vi "MC4_Sensor View Window.vi"(10 "SRV In":refnum<k5>, 11 "Sensors Config File Path":path) -> (0 "error out":errorcluster)   [LabVIEW 2009]
doc: "Save a renamed copy of this template to a location of your choice. Set \"Sensor Window Filepath\" in your System Config to point to your copy of the Sensor Window.\n\nSet \"Make All Visible\" (located just below the frame) to TRUE and run this VI directly from its own Run Arrow one time in order to make all the controls visible so that you can move controls around on the front panel. If there are sensors you will not be using, move them out of the frame off to the right.\n\nFrame should be 746x706. Check this by clicking arrow mouse over bottom right corner of frame. The window will resize to the frame at runtime.\n\nTo place IMAGE ON THE FRONT PANEL, go to Edit >> Import Picture to Clipboard (this works better in LabVIEW rather than copying to clipboard from another application). Then you can paste (Ctrl+V) the image on the front panel. It is recommended to then select your image and select Move To Back (Ctrl+Shift+J) so that sensors are on top if there is any overlap between sensors and your image.\n\n\nAuthor: Mike Schultz\n\nLogicPD, Inc\nwww.logicpd.com"
uses:
  SRV VIs/Sensors/SRV_Sensor View refs.ctl
  SRV VIs/Sensors/SRV_Sensor Config Cluster.ctl
  SRV VIs/Sensors/SRV_Sensor Analog-Digital.ctl
  SRV VIs/Sensors/SRV_Sensor Sampling Mode.ctl
  SRV VIs/Sensors/SRV_Sensor View Config Cluster.ctl
  SRV VIs/Sensors/SRV_Sensors Names.ctl
  SRV VIs/Sensors/SRV_Sensor PicoC Shared Var Type.ctl
  SRV VIs/Sensors/SRV_Sensor Config-Command Cluster.ctl
  SRV VIs/Support/SRV_Command-Data Queue Data Type.ctl
  SRV VIs/Sensors/SRV_Sensor-Value Cluster.ctl
  <vilib>/Utility/error.llb/DialogType.ctl
panel:
  in  "Make All Visible":bool
  out "Overflow Indicator":bool
  out "# elements in queue":i32
  out "Command":string
  in  "Poll":bool
  out "Boolean 32":bool
  out "Boolean 31":bool
  out "Boolean 30":bool
  out "Boolean 29":bool
  out "Boolean 28":bool
  out "Boolean 27":bool
  out "Boolean 26":bool
  out "Boolean 25":bool
  out "Boolean 24":bool
  out "Boolean 23":bool
  out "Boolean 22":bool
  out "Boolean 21":bool
  out "Boolean 20":bool
  out "Boolean 19":bool
  out "Boolean 18":bool
  out "Boolean 17":bool
  out "Boolean 16":bool
  out "Boolean 15":bool
  out "Boolean 14":bool
  out "Boolean 13":bool
  out "Boolean 12":bool
  out "Boolean 11":bool
  out "Boolean 10":bool
  out "Boolean 09":bool
  out "Boolean 08":bool
  out "Boolean 07":bool
  out "Boolean 06":bool
  out "Boolean 05":bool
  out "Boolean 04":bool
  out "Boolean 03":bool
  out "Boolean 02":bool
  out "Boolean 01":bool
  out "Numeric 08":dbl
  out "Numeric 07":dbl
  out "Numeric 06":dbl
  out "Numeric 05":dbl
  out "Numeric 04":dbl
  out "Numeric 03":dbl
  out "Numeric 02":dbl
  out "Numeric 01":dbl
  out "Meter 04":dbl(knob) scale=-1.0..0.0
  out "Meter 03":dbl(knob) scale=-1.0..0.0
  out "Meter 02":dbl(knob) scale=-1.0..0.0
  out "Meter 01":dbl(knob) scale=-1.0..0.0
  out "Gauge 04":dbl(knob) scale=-1.0..0.0
  out "Gauge 03":dbl(knob) scale=-1.0..0.0
  out "Gauge 02":dbl(knob) scale=-1.0..0.0
  out "Gauge 01":dbl(knob) scale=-1.0..0.0 scale format="%#.3g"
  # "SensorView Window"
  # "SensorPallet"
  # "SensorView Window Instructions\n\nUse the Arrow tool from the Tools Pallet to select, pull and place sensors into the SensorView Window. If you want to remove a sensor from the SensorView Window use the Arrow tool to select and pull the sensor back to the SensorPallet.\n\nTo open the Tools Pallet go to View/Tools Pallet in the standard tool bar. Be sure to close the Tools Pallet when you are finished creating your sensor dashboard.\n\n\n* BE SURE TO PLACE SENSORS BACK IN THEIR CORRECT LOCATION ON THE SENSORPALLET OR YOU WILL END UP WITH A MESS."
  # "Set to TRUE and run this VI directly from its own Run Arrow \none time in order to make all the controls visible so that \nyou can move controls around on the front panel.  If there \nare sensors you will not be using, move them out of the \nframe off to the right."
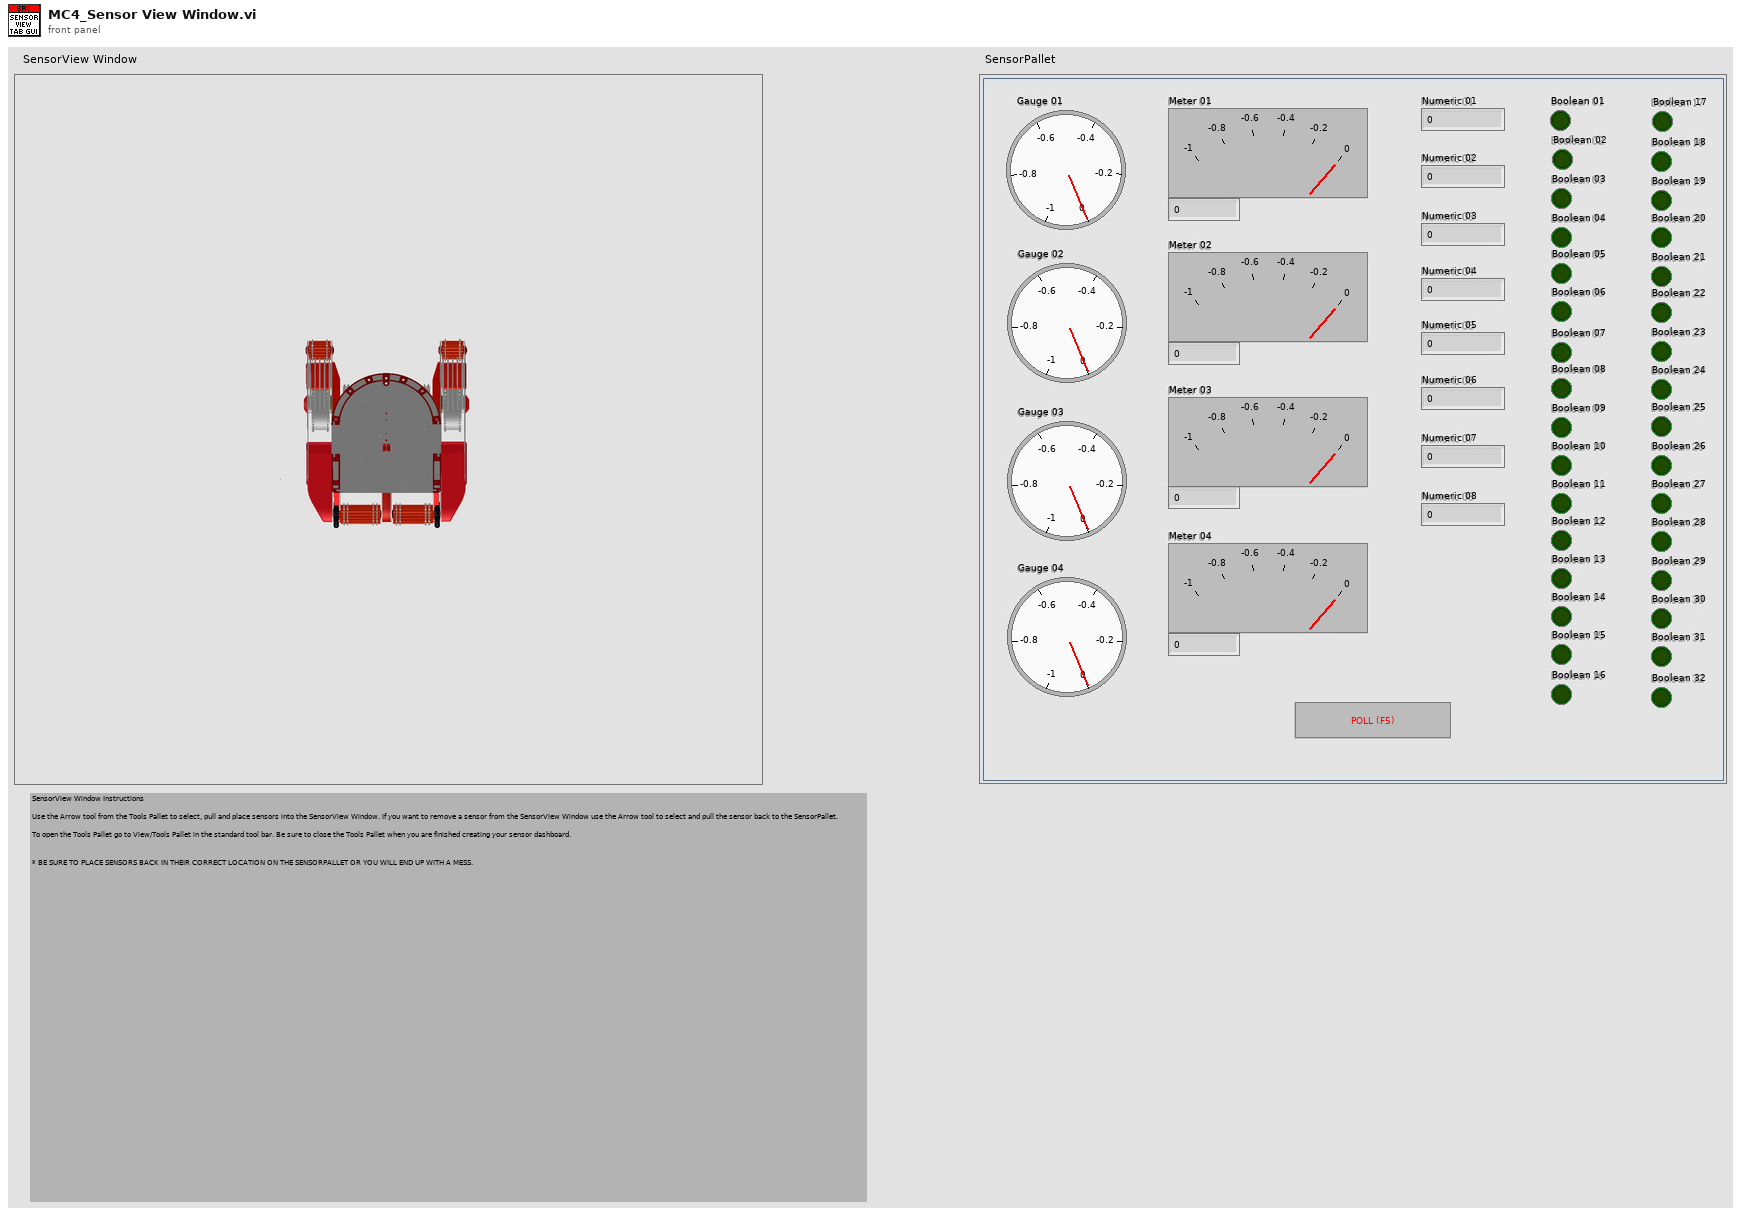
[diagram p1: front panel]
types:
  T1 = typedef "SRV_Command-Data Queue Data Type.ctl" = cluster{"Command":string, "Data":variant}
  T2 = typedef "SRV_Sensor View refs.ctl" = cluster{"Knob refs":refnum<vi>[], "Numeric refs":refnum<vi>[], "Boolean refs":refnum<vi>[]}
  T3 = typedef "SRV_Sensor Config Cluster.ctl" = cluster{"Name":string, "A/D":T4, "I2C Address":u8, "Register":u8, "Channel":u8, "Digital Mask":u8, "Units":string, "Sampling Mode":T5, "Sample Period (ms)":u32, "Formula":string, "Sensor View Config":T6, "Active":bool, "PicoC Shared Var Type":T8, "Index":u8, "Stream Multiple?":bool, "Index End":u8}
  T4 = typedef "SRV_Sensor Analog-Digital.ctl" = enum16{"Analog", "Digital", "RCMx1 Analog", "PicoC Shared"}
  T5 = typedef "SRV_Sensor Sampling Mode.ctl" = enum16{"Polled", "Streaming"}
  T6 = typedef "SRV_Sensor View Config Cluster.ctl" = cluster{"Sensor Name":T7, "Minimum":dbl, "Maximum":dbl}
  T7 = typedef "SRV_Sensors Names.ctl" = enum16{"Gauge 01", "Gauge 02", "Gauge 03", "Gauge 04", "Meter 01", "Meter 02", "Meter 03", "Meter 04", "Numeric 01", "Numeric 02", "Numeric 03", "Numeric 04", "Numeric 05", "Numeric 06", "Numeric 07", "Numeric 08", "Boolean 01", "Boolean 02", "Boolean 03", "Boolean 04", "Boolean 05", "Boolean 06", "Boolean 07", "Boolean 08", "Boolean 09", "Boolean 10", "Boolean 11", "Boolean 12", "Boolean 13", "Boolean 14", "Boolean 15", "Boolean 16", "Boolean 17", "Boolean 18", "Boolean 19", "Boolean 20", "Boolean 21", "Boolean 22", "Boolean 23", "Boolean 24", "Boolean 25", "Boolean 26", "Boolean 27", "Boolean 28", "Boolean 29", "Boolean 30", "Boolean 31", "Boolean 32"}
  T8 = typedef "SRV_Sensor PicoC Shared Var Type.ctl" = enum16{"String", "Integer", "Float"}
  T9 = typedef "SRV_Sensor Config-Command Cluster.ctl" = cluster{"Sensor Config":T3, "Command":string, "Constant Command":string}
  T10 = cluster{"user event":refnum<user-event>, "Version":string, "Sensor View refs":T2, "This VI ref":refnum<vi>, "Sensors Config File Path":path, "Sensors Config":T3[], "SRV ref":refnum<k5>, "Streaming Cfg-Cmds":T9[], "Polled Cfg-Cmds":T9[], "Off Cfg-Cmds":T9[], "Streaming Constant Commands":string[], "Polled Constant Commands":string[], "Make All Visible":bool}
  T11 = typedef "SRV_Sensor-Value Cluster.ctl" = cluster{"Sensor Name":T7, "Value":dbl}
  T12 = typedef "DialogType.ctl" = u16
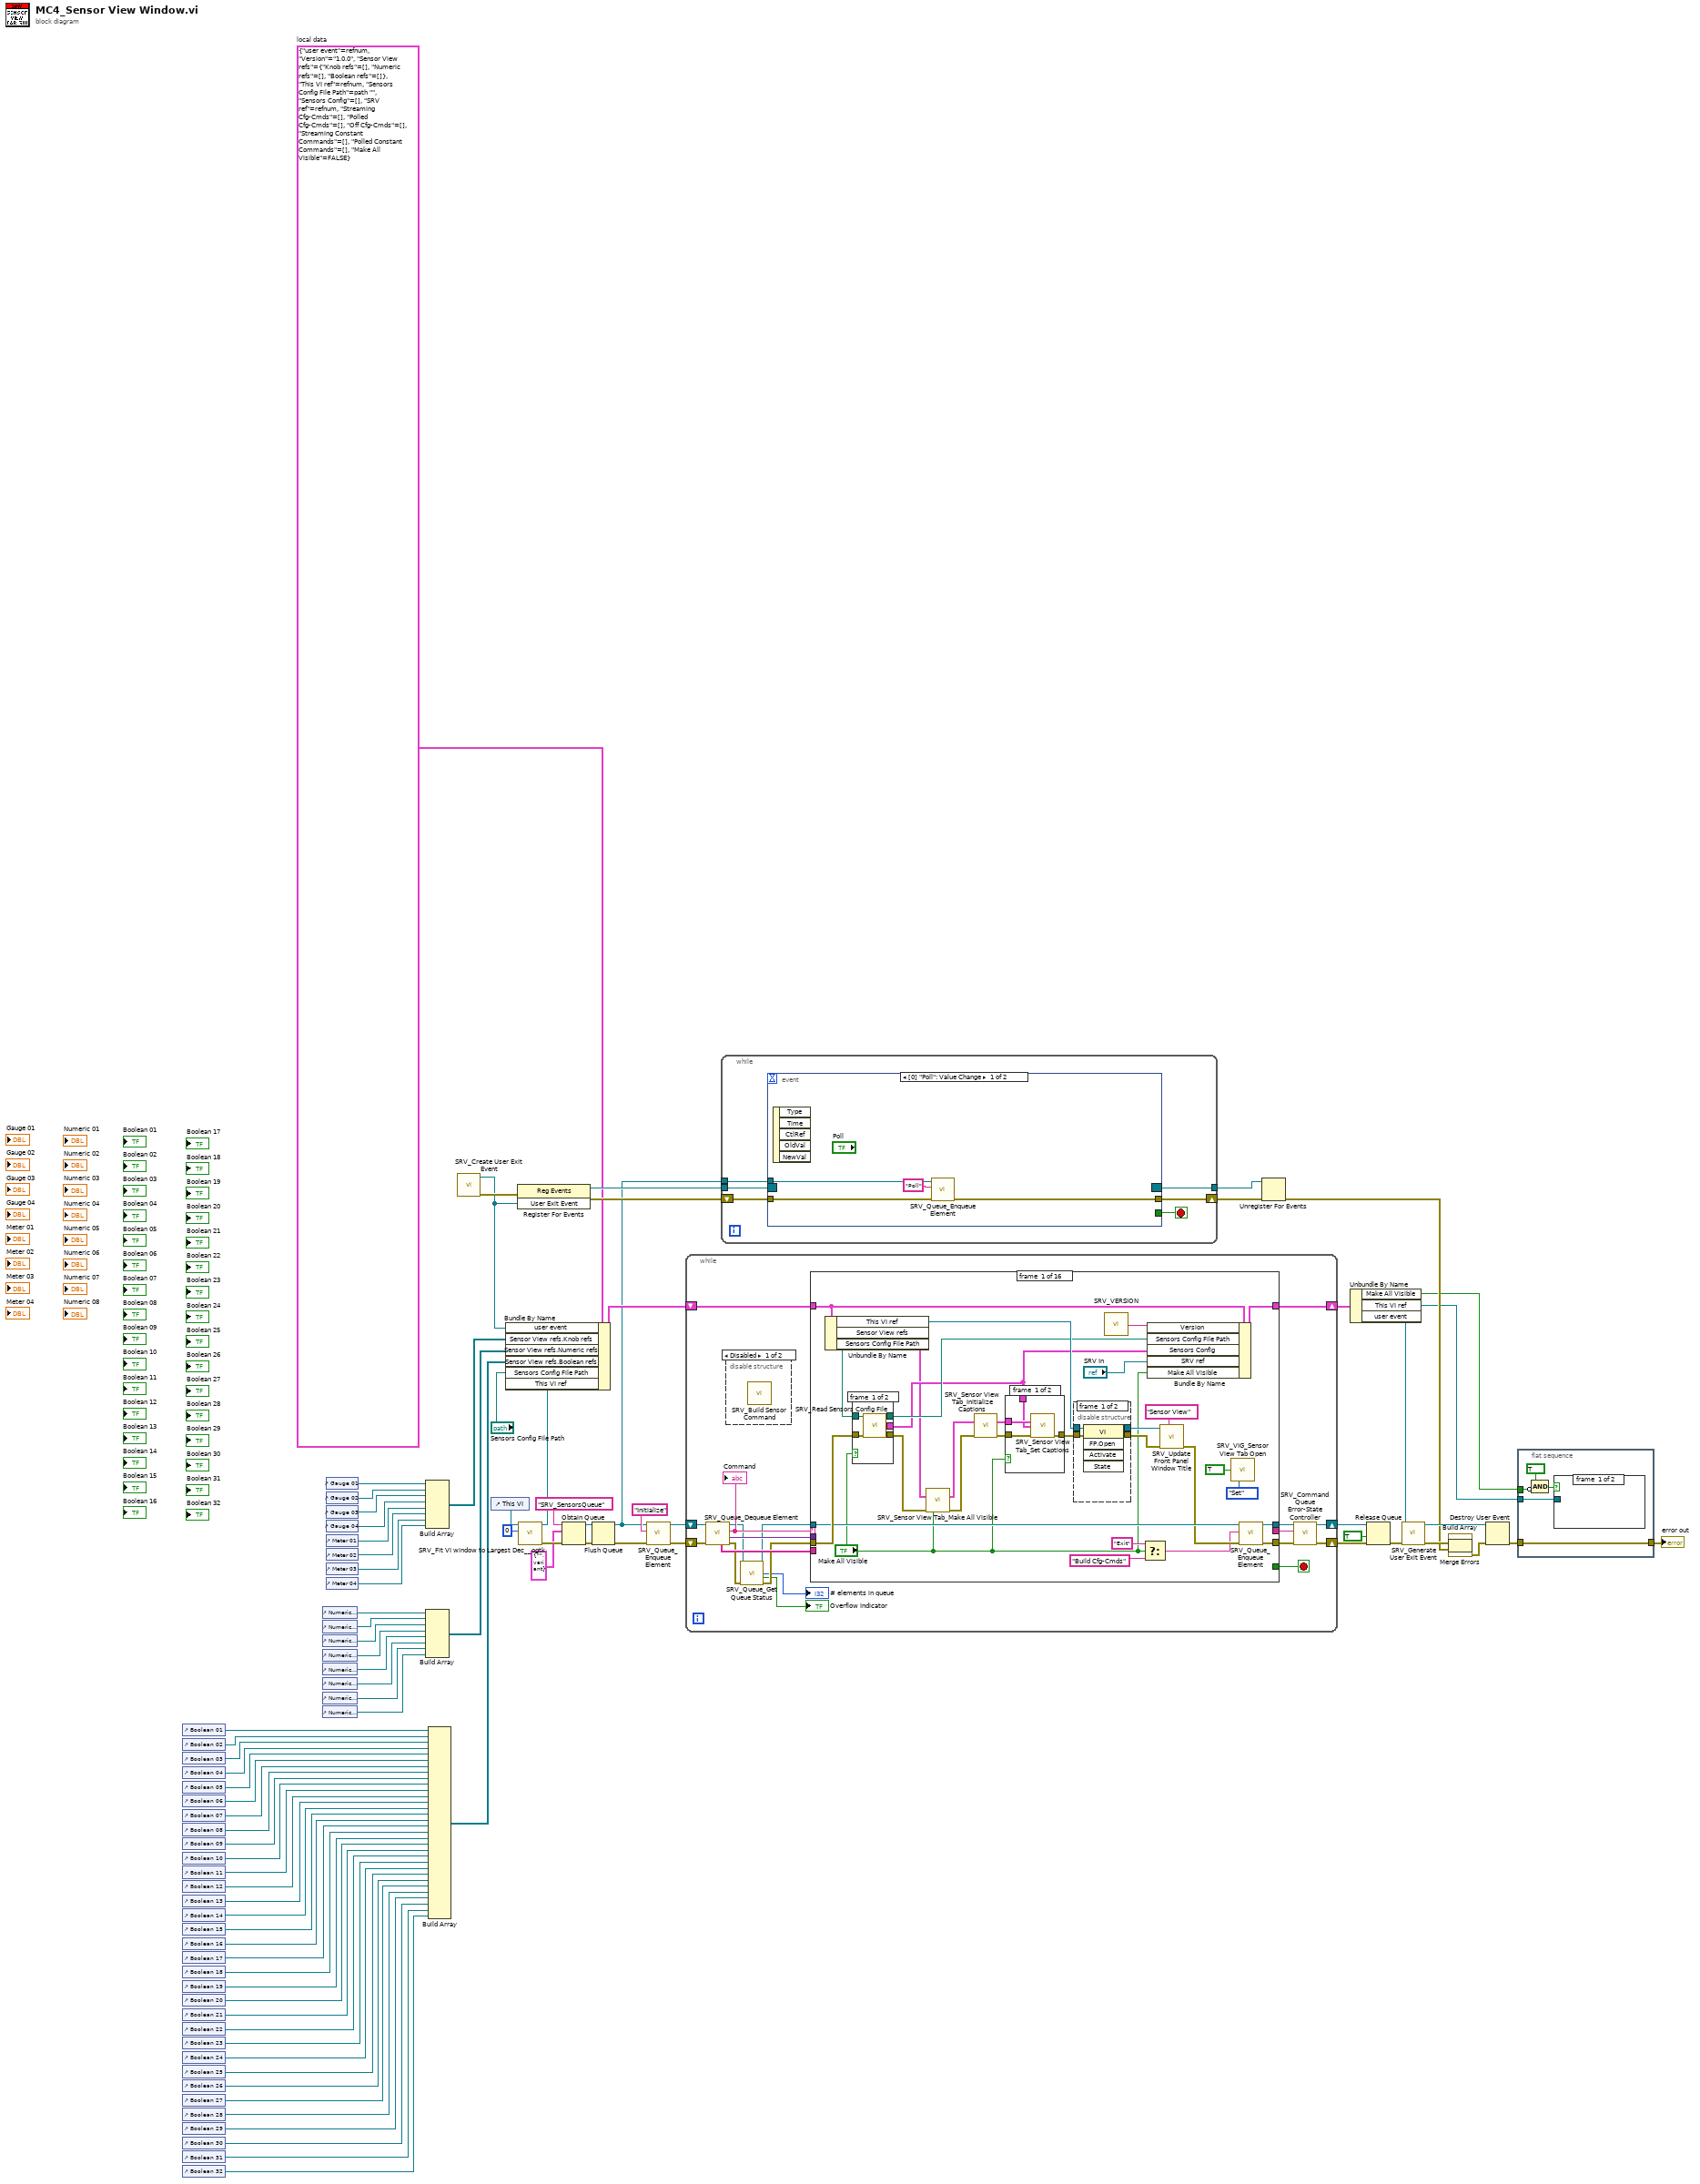
[diagram p0: block diagram]
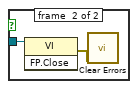
[diagram p2: hidden frame]
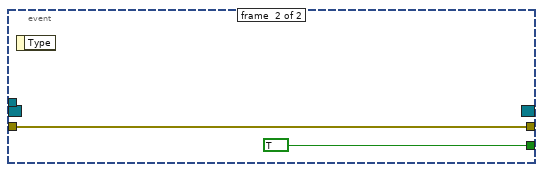
[diagram p3: hidden frame]
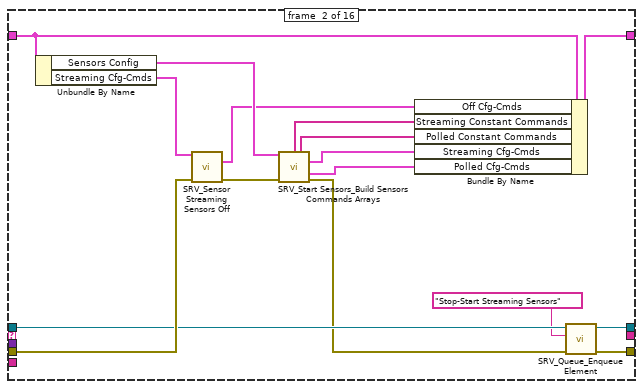
[diagram p8: hidden frame]
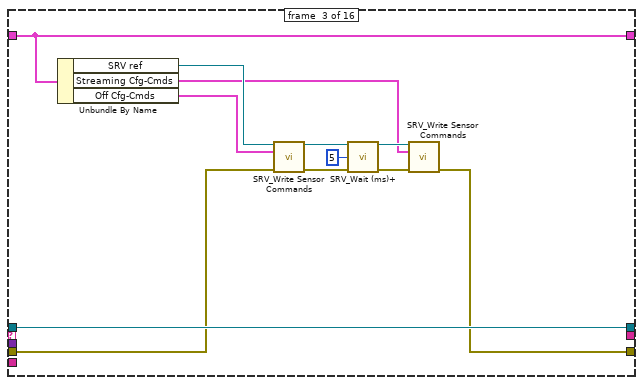
[diagram p9: hidden frame]
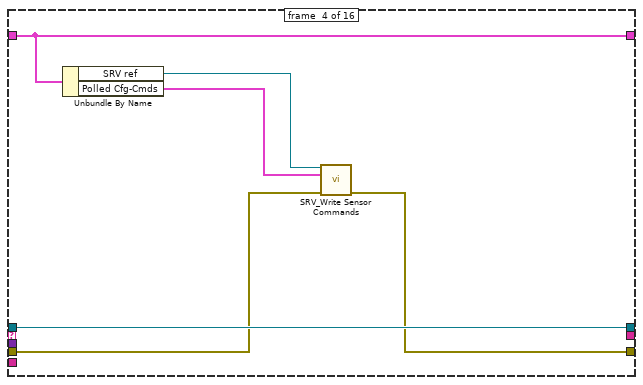
[diagram p10: hidden frame]
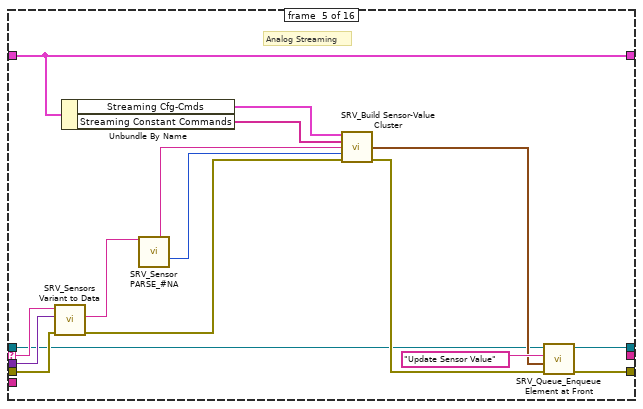
[diagram p11: hidden frame]
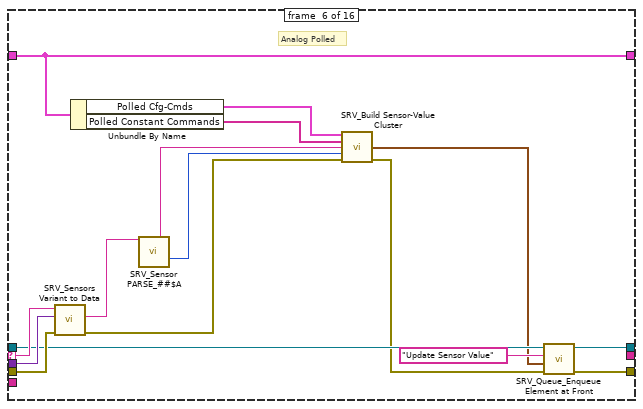
[diagram p12: hidden frame]
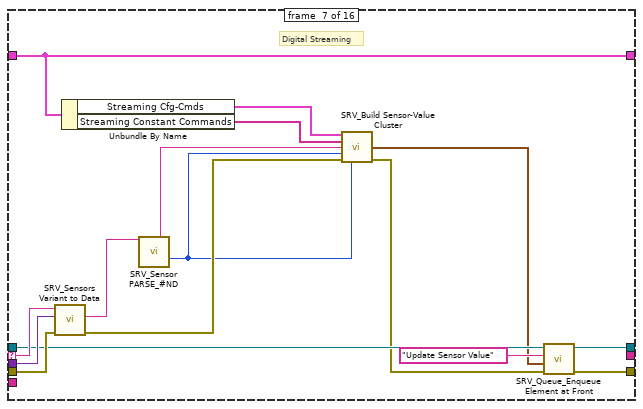
[diagram p13: hidden frame]
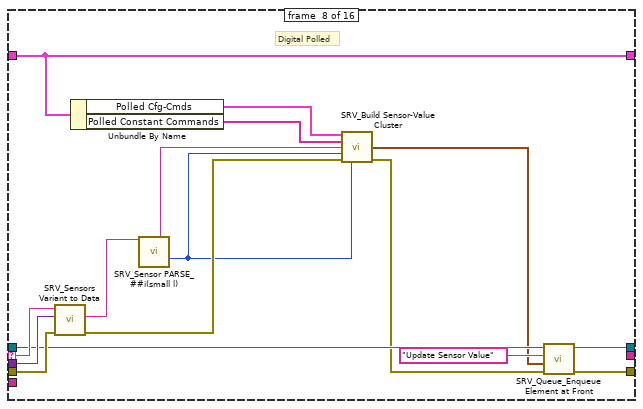
[diagram p14: hidden frame]
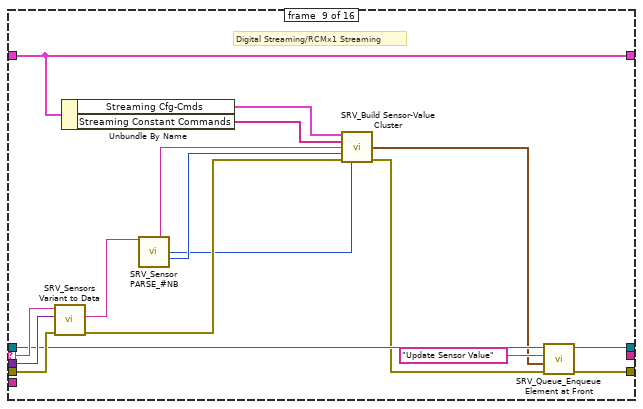
[diagram p15: hidden frame]
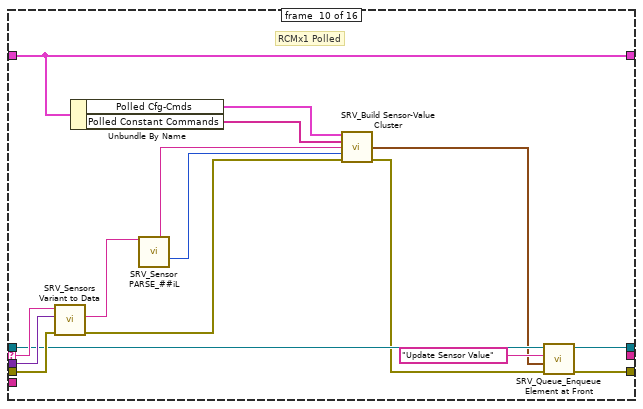
[diagram p16: hidden frame]
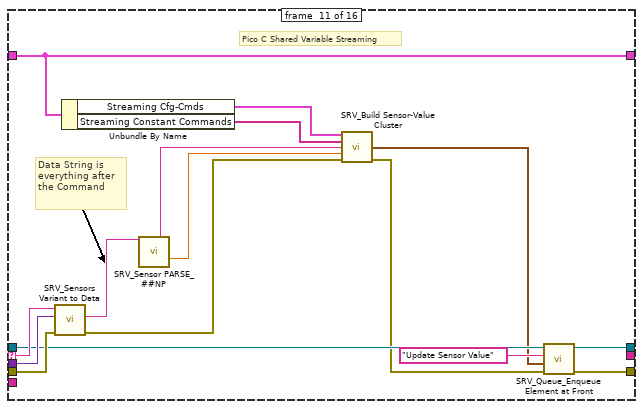
[diagram p17: hidden frame]
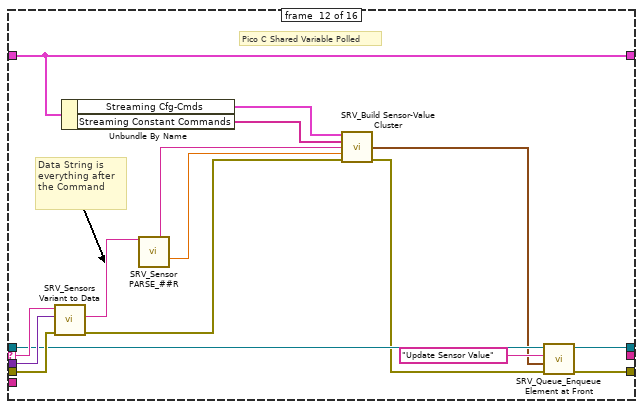
[diagram p18: hidden frame]
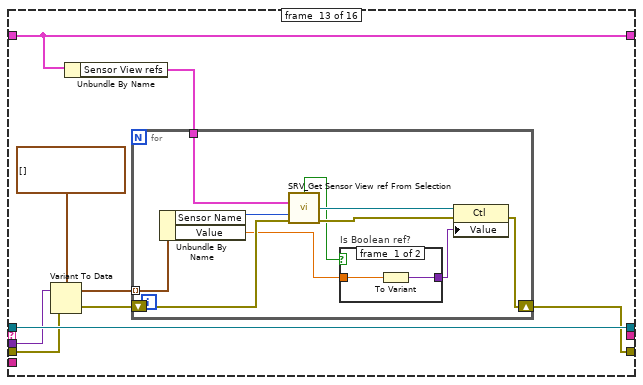
[diagram p19: hidden frame]
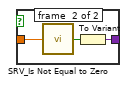
[diagram p20: hidden frame]
diagram:
  w82 = T10 {"user event"=refnum, "Version"="1.0.0", "Sensor View refs"={"Knob refs"=[], "Numeric refs"=[], "Boolean refs"=[]}, "This VI ref"=refnum, "Sensors Config File Path"=path "", "Sensors Config"=[], "SRV ref"=refnum, "Streaming Cfg-Cmds"=[], "Polled Cfg-Cmds"=[], "Off Cfg-Cmds"=[], "Streaming Constant Commands"=[], "Polled Constant Commands"=[], "Make All Visible"=FALSE}  # local data
  n1 = control-ref of="Boolean 01"() -> (w49:refnum<vi>)
  n2 = control-ref of="Boolean 02"() -> (w48:refnum<vi>)
  n3 = control-ref of="Boolean 03"() -> (w47:refnum<vi>)
  n4 = control-ref of="Boolean 04"() -> (w46:refnum<vi>)
  n5 = control-ref of="Boolean 05"() -> (w45:refnum<vi>)
  n6 = control-ref of="Boolean 06"() -> (w44:refnum<vi>)
  n7 = control-ref of="Boolean 07"() -> (w43:refnum<vi>)
  n8 = control-ref of="Boolean 08"() -> (w42:refnum<vi>)
  n9 = control-ref of="Boolean 09"() -> (w41:refnum<vi>)
  n10 = control-ref of="Boolean 10"() -> (w40:refnum<vi>)
  n11 = control-ref of="Boolean 11"() -> (w39:refnum<vi>)
  n12 = control-ref of="Boolean 12"() -> (w38:refnum<vi>)
  n13 = control-ref of="Boolean 13"() -> (w37:refnum<vi>)
  n14 = control-ref of="Boolean 14"() -> (w36:refnum<vi>)
  n15 = control-ref of="Boolean 15"() -> (w35:refnum<vi>)
  n16 = control-ref of="Boolean 16"() -> (w34:refnum<vi>)
  n17 = control-ref of="Boolean 17"() -> (w33:refnum<vi>)
  n18 = control-ref of="Boolean 18"() -> (w32:refnum<vi>)
  n19 = control-ref of="Boolean 19"() -> (w31:refnum<vi>)
  n20 = control-ref of="Boolean 20"() -> (w30:refnum<vi>)
  n21 = control-ref of="Boolean 21"() -> (w29:refnum<vi>)
  n22 = control-ref of="Boolean 22"() -> (w28:refnum<vi>)
  n23 = control-ref of="Boolean 23"() -> (w27:refnum<vi>)
  n24 = control-ref of="Boolean 24"() -> (w26:refnum<vi>)
  n25 = control-ref of="Boolean 25"() -> (w25:refnum<vi>)
  n26 = control-ref of="Boolean 26"() -> (w24:refnum<vi>)
  n27 = control-ref of="Boolean 27"() -> (w23:refnum<vi>)
  n28 = control-ref of="Boolean 28"() -> (w22:refnum<vi>)
  n29 = control-ref of="Boolean 29"() -> (w21:refnum<vi>)
  n30 = control-ref of="Boolean 30"() -> (w20:refnum<vi>)
  n31 = control-ref of="Boolean 31"() -> (w19:refnum<vi>)
  n32 = control-ref of="Boolean 32"() -> (w18:refnum<vi>)
  n33 = control-ref of="Numeric 01"() -> (w57:refnum<vi>)
  n34 = control-ref of="Numeric 02"() -> (w56:refnum<vi>)
  n35 = control-ref of="Numeric 03"() -> (w55:refnum<vi>)
  n36 = control-ref of="Numeric 04"() -> (w54:refnum<vi>)
  n37 = control-ref of="Numeric 05"() -> (w53:refnum<vi>)
  n38 = control-ref of="Numeric 06"() -> (w52:refnum<vi>)
  n39 = control-ref of="Numeric 07"() -> (w51:refnum<vi>)
  n40 = control-ref of="Numeric 08"() -> (w50:refnum<vi>)
  n41 = control-ref of="Gauge 01"() -> (w65:refnum<vi>)
  n42 = control-ref of="Gauge 02"() -> (w64:refnum<vi>)
  n43 = control-ref of="Gauge 03"() -> (w63:refnum<vi>)
  n44 = control-ref of="Gauge 04"() -> (w62:refnum<vi>)
  n45 = control-ref of="Meter 01"() -> (w61:refnum<vi>)
  n46 = control-ref of="Meter 02"() -> (w60:refnum<vi>)
  n47 = control-ref of="Meter 03"() -> (w59:refnum<vi>)
  n48 = control-ref of="Meter 04"() -> (w58:refnum<vi>)
  n49 = Build Array(w65, w64, w63, w62, w61, w60, w59, w58) -> (w12:refnum<vi>[])
  n50 = Build Array(w57, w56, w55, w54, w53, w52, w51, w50) -> (w13:refnum<vi>[])
  n51 = Build Array(w49, w48, w47, w46, w45, w44, w43, w42, w41, w40, w39, w38, w37, w36, w35, w34, w33, w32, w31, w30, w29, w28, w27, w26, w25, w24, w23, w22, w21, w20, w19, w18) -> (w14:refnum<vi>[])
  n52 = call "SRV_Create User Exit Event.vi"() -> ("error out"=w73:errorcluster, "User Exit Event"=w72:refnum<user-event>)  [unwired: 10 in]
  n53 = control-ref of="This VI"() -> (w3:refnum<vi>)
  n54 = register-events(error in=w73, w72) -> (reference out=w88:refnum<event-registration>, error out=w87:errorcluster)  [unwired: 1 in]
  n55 = call "SRV_Fit VI window to Largest Dec__ogtk.vi"("border spacing (2 px)"=0, "VI Ref (calling VI)"=w3) -> ("error out"=w68:errorcluster, "dup VI Ref"=w11:refnum<vi>)  [unwired: 4 in]
  n56 = Bundle By Name(cluster=w82, "user event"=w72, "Sensor View refs.Knob refs"=w12, "Sensor View refs.Numeric refs"=w13, "Sensor View refs.Boolean refs"=w14, "Sensors Config File Path"="Sensors Config File Path", "This VI ref"=w11) -> (w81:T10)
  n57 = Obtain Queue(name (unnamed)="SRV_SensorsQueue", element data type=T1 {"Command"="", "Data"=variant} ("Queue Data Type"), error in (no error)=w68) -> (queue out=w5:refnum<queue>, error out=w7:errorcluster)  [unwired: 2 in, 1 out]
  n58 = Flush Queue(queue=w5, error in (no error)=w7) -> (queue out=w4:refnum<queue>, error out=w6:errorcluster)  [unwired: 1 out]
  n59 = call "SRV_Queue_Enqueue Element.vi"("error in (no error)"=w6, "Command"="Initialize", "Command-Data Queue"=w4) -> ("error out"=w66:errorcluster, "Command-Data Queue out"=w69:refnum<queue>)  [unwired: 6 in, 1 out]
  n60 = while {
    shift-right: [w103] -> w84
    shift-left: w66 -> [w107]
    shift-right: [w101] -> w83
    shift-left: w69 -> [w106]
    shift-right: [w95] -> w80
    shift-left: w81 -> [w96]
    stop <- w97 stop-if-true
    n61 = call "SRV_Queue_Dequeue Element.vi"("error in (no error)"=w107, "Command-Data Queue"=w106) -> ("error out"=w94:errorcluster, "Data"=w100:variant, "Command"=w105:string, "Command-Data Queue out"=w92:refnum<queue>, "Command History"=w99:string[])  [unwired: 4 in, 1 out]
    "Command" <- w105
    n62 = disable-structure shown="Disabled" {
      frame #0 {
        n63 = call "SRV_Build Sensor Command.vi"() -> ()  [unwired: 9 in, 7 out]
      }
      frame #1 {
      }
    }
    n64 = call "SRV_Queue_Get Queue Status.vi"("Command-Data Queue"=w92, "error in (no error)"=w94) -> ("Command-Data Queue out"=w91:refnum<queue>, "# elements in queue"=→"# elements in queue":i32, "Overflow Indicator"=→"Overflow Indicator":bool, "error out"=w93:errorcluster)  [unwired: 10 in]
    n65 = case shown="\"Initialize\"" w105 {
      selector: w105 -> [_ _ _ _ w202 w218 w234 w250 w267 w283 w299 w315 _ w345 _ _]
      tunnel: w93 -> [w135 w164 w179 w183 w189 w217 w233 w249 w266 w282 w298 w314 w324 w343 w352 w359]
      tunnel: [w125 w159 w174 w182 w193 w206 w223 w239 w256 w271 w287 w303 w318 w342 w349 w358] -> w104
      tunnel: w91 -> [w127 w161 w180 w187 w188 w209 w226 w242 w259 w274 w290 w306 w325 w347 w356 w369]
      tunnel: [w126 w160 w180 w187 w195 w208 w225 w241 w258 w273 w289 w305 w325 w347 w356 w369] -> w102
      tunnel: w100 -> [_ _ _ _ w203 w219 w235 w251 w268 w284 w300 w316 w323 _ _ _]
      tunnel: w99 -> [_ _ _ _ _ _ _ _ _ _ _ _ _ _ w355 _]
      tunnel: [_ _ _ _ _ _ _ _ _ _ _ _ _ _ "Exit" ("Error Command") _] -> w98
      tunnel: [_ _ _ _ _ _ _ _ _ _ _ _ _ _ _ TRUE] -> w97
      tunnel: w96 -> [w114 w169 w181 w186 w200 w215 w231 w247 w264 w280 w296 w312 w322 w344 w353 w365]
      tunnel: [w136 w168 w181 w186 w200 w215 w231 w247 w264 w280 w296 w312 w322 w344 w353 w365] -> w95
      frame #0 {
        n66 = Unbundle By Name(w114) -> ("This VI ref"=w132:refnum<vi>, "Sensor View refs"=w113:T2, "Sensors Config File Path"=w129:path)
        n67 = case shown="False" "Make All Visible" {
          tunnel: w135 -> [w147 w148]
          tunnel: [w146 w149] -> w130
          tunnel: w129 -> [w145 w149]
          tunnel: [w144 _] -> w128
          tunnel: [w143 w148] -> w116
          frame #0 {
            n68 = call "SRV_Read Sensors Config File.vi"("Sensors Config File Path"=w145, "error in (no error)"=w147) -> ("Sensors Config File Path out"=w146:path, "Sensors Config"=w144:T3[], "error out"=w143:errorcluster)  [unwired: 10 in, 1 out]
          }
          frame #1 {
          }
        }
        n69 = call "SRV_Sensor View Tab_Make All Visible.vi"("Sensor View refs"=w113, "error in (no error)"=w116, "Make All Visible?"="Make All Visible") -> ("Sensor View refs dup"=w112:T2, "error out"=w115:errorcluster)  [unwired: 11 in]
        n70 = call "SRV_Sensor View Tab_Initialize Captions.vi"("Sensor View refs"=w112, "error in (no error)"=w115) -> ("Sensor View refs dup"=w133:T2, "error out"=w134:errorcluster)  [unwired: 12 in]
        n71 = case shown="False" "Make All Visible" {
          tunnel: w134 -> [w153 w154]
          tunnel: w133 -> [w152 _]
          tunnel: [w151 w154] -> w131
          tunnel: w128 -> [w150 _]
          frame #0 {
            n72 = call "SRV_Sensor View Tab_Set Captions.vi"("Sensor View refs"=w152, "Sensors Config"=w150, "error in (no error)"=w153) -> ("error out"=w151:errorcluster)  [unwired: 11 in, 1 out]
          }
          frame #1 {
          }
        }
        n73 = disable-structure shown="Enabled" {
          disable-tunnel: w132 -> [w140 w142]
          disable-tunnel: w131 -> [w139 w141]
          disable-tunnel: [w138 w141] -> w122
          disable-tunnel: [w137 w142] -> w121
          frame #0 {
            n74 = invoke class="VI" method="FP.Open"(reference=w140, error in=w139) -> (reference out=w137:refnum<vi>, error out=w138:errorcluster)  [unwired: 3 in, 3 out]
          }
          frame #1 {
          }
        }
        n75 = call "SRV_VERSION.vi"() -> ("SRV Version"=w123:string)
        n76 = Select(t="Exit", s="Make All Visible", f="Build Cfg-Cmds" ("Command")) -> (s? t:f=w111:string)
        n77 = Bundle By Name(cluster=w114, "Version"=w123, "Sensors Config File Path"=w130, "Sensors Config"=w128, "SRV ref"="SRV In", "Make All Visible"="Make All Visible") -> (w136:T10)
        n78 = call "SRV_Update Front Panel Window Title.vi"("Window Title Override String"="Sensor View", "error in (no error)"=w122, "VI ref"=w121) -> ("error out"=w120:errorcluster)  [unwired: 7 in, 1 out]
        n79 = call "SRV_VIG_Sensor View Tab Open.vi"("Sensor View Tab Open"=TRUE, "Method (Get)"=enum16{"Get", "Set"}."Set") -> ()  [unwired: 12 in, 2 out]
        n80 = call "SRV_Queue_Enqueue Element.vi"("error in (no error)"=w120, "Command"=w111, "Command-Data Queue"=w127) -> ("error out"=w125:errorcluster, "Command-Data Queue out"=w126:refnum<queue>)  [unwired: 6 in, 1 out]
      }
      frame #1 {
        n81 = Unbundle By Name(w169) -> ("Sensors Config"=w170:T3[], "Streaming Cfg-Cmds"=w165:T9[])
        n82 = call "SRV_Sensor Streaming Sensors Off.vi"("Previous Streaming Cfg-Cmds"=w165, "error in (no error)"=w164) -> ("Streaming Cfg-Cmds OFF"=w162:T9[], "error out"=w163:errorcluster)  [unwired: 12 in]
        n83 = call "SRV_Start Sensors_Build Sensors Commands Arrays.vi"("Sensors Config"=w170, "error in (no error)"=w163) -> ("Streaming Constant Commands"=w156:string[], "Polled Constant Commands"=w155:string[], "Active Streaming Cfg-Commands"=w167:T9[], "Active Polled Cfg-Commands"=w166:T9[], "error out"=w158:errorcluster)  [unwired: 9 in]
        n84 = Bundle By Name(cluster=w169, "Off Cfg-Cmds"=w162, "Streaming Constant Commands"=w156, "Polled Constant Commands"=w155, "Streaming Cfg-Cmds"=w167, "Polled Cfg-Cmds"=w166) -> (w168:T10)
        n85 = call "SRV_Queue_Enqueue Element.vi"("error in (no error)"=w158, "Command"="Stop-Start Streaming Sensors", "Command-Data Queue"=w161) -> ("error out"=w159:errorcluster, "Command-Data Queue out"=w160:refnum<queue>)  [unwired: 6 in, 1 out]
      }
      frame #2 {
        n86 = Unbundle By Name(w181) -> ("SRV ref"=w178:refnum<k5>, "Streaming Cfg-Cmds"=w175:T9[], "Off Cfg-Cmds"=w177:T9[])
        n87 = call "SRV_Write Sensor Commands.vi"("SRV In"=w178, "Sensor Cfg-Commands"=w177, "error in (no error)"=w179) -> ("SRV out"=w176:refnum<k5>, "error out"=w173:errorcluster)  [unwired: 11 in]
        n88 = call "SRV_Wait (ms)+.vi"("milliseconds to wait"=u32 5, "error in (no error)"=w173) -> ("error out"=w172:errorcluster)  [unwired: 12 in, 1 out]
        n89 = call "SRV_Write Sensor Commands.vi"("SRV In"=w176, "Sensor Cfg-Commands"=w175, "error in (no error)"=w172) -> ("error out"=w174:errorcluster)  [unwired: 11 in, 1 out]
      }
      frame #3 {
        n90 = Unbundle By Name(w186) -> ("SRV ref"=w184:refnum<k5>, "Polled Cfg-Cmds"=w185:T9[])
        n91 = call "SRV_Write Sensor Commands.vi"("SRV In"=w184, "Sensor Cfg-Commands"=w185, "error in (no error)"=w183) -> ("error out"=w182:errorcluster)  [unwired: 11 in, 1 out]
      }
      frame #4 {
        # "Analog Streaming"
        n92 = call "SRV_Sensors Variant to Data.vi"("error in (no error)"=w189, "Data"=w203, "Command"=w202) -> ("error out"=w190:errorcluster, "Data String"=w201:string)  [unwired: 7 in]
        n93 = Unbundle By Name(w200) -> ("Streaming Cfg-Cmds"=w199:T9[], "Streaming Constant Commands"=w198:string[])
        n94 = call "SRV_Sensor PARSE_#NA.vi"("Return Data"=w201) -> ("Constant Command"=w197:string, "Value"=w196:u16)  [unwired: 13 in]
        n95 = call "SRV_Build Sensor-Value Cluster.vi"("Cfg-Cmds"=w199, "Constant Commands"=w198, "Constant Command"=w197, "Value"=w196, "error in (no error)"=w190) -> ("Array of Sensor-Value Cluster"=w191:T11[], "error out"=w194:errorcluster)  [unwired: 9 in]
        n96 = call "SRV_Queue_Enqueue Element at Front.vi"("error in (no error)"=w194, "Data"=w191, "Command"="Update Sensor Value", "Command-Data Queue"=w188) -> ("error out"=w193:errorcluster, "Command-Data Queue out"=w195:refnum<queue>)  [unwired: 5 in, 1 out]
      }
      frame #5 {
        # "Analog Polled"
        n97 = call "SRV_Sensors Variant to Data.vi"("error in (no error)"=w217, "Data"=w219, "Command"=w218) -> ("error out"=w210:errorcluster, "Data String"=w216:string)  [unwired: 7 in]
        n98 = Unbundle By Name(w215) -> ("Polled Cfg-Cmds"=w214:T9[], "Polled Constant Commands"=w213:string[])
        n99 = call "SRV_Sensor PARSE_##$A.vi"("Return Data"=w216) -> ("Constant Command"=w212:string, "Value"=w211:u16)  [unwired: 13 in]
        n100 = call "SRV_Build Sensor-Value Cluster.vi"("Cfg-Cmds"=w214, "Constant Commands"=w213, "Constant Command"=w212, "Value"=w211, "error in (no error)"=w210) -> ("Array of Sensor-Value Cluster"=w204:T11[], "error out"=w207:errorcluster)  [unwired: 9 in]
        n101 = call "SRV_Queue_Enqueue Element at Front.vi"("error in (no error)"=w207, "Data"=w204, "Command"="Update Sensor Value", "Command-Data Queue"=w209) -> ("error out"=w206:errorcluster, "Command-Data Queue out"=w208:refnum<queue>)  [unwired: 5 in, 1 out]
      }
      frame #6 {
        # "Digital Streaming"
        n102 = call "SRV_Sensors Variant to Data.vi"("error in (no error)"=w233, "Data"=w235, "Command"=w234) -> ("error out"=w227:errorcluster, "Data String"=w232:string)  [unwired: 7 in]
        n103 = Unbundle By Name(w231) -> ("Streaming Cfg-Cmds"=w230:T9[], "Streaming Constant Commands"=w229:string[])
        n104 = call "SRV_Sensor PARSE_#ND.vi"("Return Data"=w232) -> ("Constant Command"=w228:string, "Value"=w220:u8)  [unwired: 13 in]
        n105 = call "SRV_Build Sensor-Value Cluster.vi"("Cfg-Cmds"=w230, "Constant Commands"=w229, "Constant Command"=w228, "Value"=w220, "error in (no error)"=w227, "Value (U8)"=w220) -> ("Array of Sensor-Value Cluster"=w221:T11[], "error out"=w224:errorcluster)  [unwired: 8 in]
        n106 = call "SRV_Queue_Enqueue Element at Front.vi"("error in (no error)"=w224, "Data"=w221, "Command"="Update Sensor Value", "Command-Data Queue"=w226) -> ("error out"=w223:errorcluster, "Command-Data Queue out"=w225:refnum<queue>)  [unwired: 5 in, 1 out]
      }
      frame #7 {
        # "Digital Polled"
        n107 = call "SRV_Sensors Variant to Data.vi"("error in (no error)"=w249, "Data"=w251, "Command"=w250) -> ("error out"=w243:errorcluster, "Data String"=w248:string)  [unwired: 7 in]
        n108 = Unbundle By Name(w247) -> ("Polled Cfg-Cmds"=w246:T9[], "Polled Constant Commands"=w245:string[])
        n109 = call "SRV_Sensor PARSE_##i(small l).vi"("Return Data"=w248) -> ("Constant Command"=w244:string, "Value"=w236:u8)  [unwired: 13 in]
        n110 = call "SRV_Build Sensor-Value Cluster.vi"("Cfg-Cmds"=w246, "Constant Commands"=w245, "Constant Command"=w244, "Value"=w236, "error in (no error)"=w243, "Value (U8)"=w236) -> ("Array of Sensor-Value Cluster"=w237:T11[], "error out"=w240:errorcluster)  [unwired: 8 in]
        n111 = call "SRV_Queue_Enqueue Element at Front.vi"("error in (no error)"=w240, "Data"=w237, "Command"="Update Sensor Value", "Command-Data Queue"=w242) -> ("error out"=w239:errorcluster, "Command-Data Queue out"=w241:refnum<queue>)  [unwired: 5 in, 1 out]
      }
      frame #8 {
        # "Digital Streaming/RCMx1 Streaming"
        n112 = call "SRV_Sensors Variant to Data.vi"("error in (no error)"=w266, "Data"=w268, "Command"=w267) -> ("error out"=w260:errorcluster, "Data String"=w265:string)  [unwired: 7 in]
        n113 = Unbundle By Name(w264) -> ("Streaming Cfg-Cmds"=w263:T9[], "Streaming Constant Commands"=w262:string[])
        n114 = call "SRV_Sensor PARSE_#NB.vi"("Return Data"=w265) -> ("Constant Command"=w261:string, "Value (U8)"=w252:u8, "Value"=w253:u16)  [unwired: 12 in]
        n115 = call "SRV_Build Sensor-Value Cluster.vi"("Cfg-Cmds"=w263, "Constant Commands"=w262, "Constant Command"=w261, "Value"=w253, "error in (no error)"=w260, "Value (U8)"=w252) -> ("Array of Sensor-Value Cluster"=w254:T11[], "error out"=w257:errorcluster)  [unwired: 8 in]
        n116 = call "SRV_Queue_Enqueue Element at Front.vi"("error in (no error)"=w257, "Data"=w254, "Command"="Update Sensor Value", "Command-Data Queue"=w259) -> ("error out"=w256:errorcluster, "Command-Data Queue out"=w258:refnum<queue>)  [unwired: 5 in, 1 out]
      }
      frame #9 {
        # "RCMx1 Polled"
        n117 = call "SRV_Sensors Variant to Data.vi"("error in (no error)"=w282, "Data"=w284, "Command"=w283) -> ("error out"=w275:errorcluster, "Data String"=w281:string)  [unwired: 7 in]
        n118 = Unbundle By Name(w280) -> ("Polled Cfg-Cmds"=w279:T9[], "Polled Constant Commands"=w278:string[])
        n119 = call "SRV_Sensor PARSE_##iL.vi"("Return Data"=w281) -> ("Constant Command"=w277:string, "Value"=w276:u16)  [unwired: 13 in]
        n120 = call "SRV_Build Sensor-Value Cluster.vi"("Cfg-Cmds"=w279, "Constant Commands"=w278, "Constant Command"=w277, "Value"=w276, "error in (no error)"=w275) -> ("Array of Sensor-Value Cluster"=w269:T11[], "error out"=w272:errorcluster)  [unwired: 9 in]
        n121 = call "SRV_Queue_Enqueue Element at Front.vi"("error in (no error)"=w272, "Data"=w269, "Command"="Update Sensor Value", "Command-Data Queue"=w274) -> ("error out"=w271:errorcluster, "Command-Data Queue out"=w273:refnum<queue>)  [unwired: 5 in, 1 out]
      }
      frame #10 {
        # "Data String is everything after the Command"
        # "Pico C Shared Variable Streaming"
        n122 = call "SRV_Sensors Variant to Data.vi"("error in (no error)"=w298, "Data"=w300, "Command"=w299) -> ("error out"=w291:errorcluster, "Data String"=w297:string)  [unwired: 7 in]
        n123 = Unbundle By Name(w296) -> ("Streaming Cfg-Cmds"=w295:T9[], "Streaming Constant Commands"=w294:string[])
        n124 = call "SRV_Sensor PARSE_##NP.vi"("Return Data"=w297) -> ("Constant Command"=w293:string, "Value"=w292:dbl)  [unwired: 13 in]
        n125 = call "SRV_Build Sensor-Value Cluster.vi"("Cfg-Cmds"=w295, "Constant Commands"=w294, "Constant Command"=w293, "Value"=w292, "error in (no error)"=w291) -> ("Array of Sensor-Value Cluster"=w285:T11[], "error out"=w288:errorcluster)  [unwired: 9 in]
        n126 = call "SRV_Queue_Enqueue Element at Front.vi"("error in (no error)"=w288, "Data"=w285, "Command"="Update Sensor Value", "Command-Data Queue"=w290) -> ("error out"=w287:errorcluster, "Command-Data Queue out"=w289:refnum<queue>)  [unwired: 5 in, 1 out]
      }
      frame #11 {
        # "Data String is everything after the Command"
        # "Pico C Shared Variable Polled"
        n127 = call "SRV_Sensors Variant to Data.vi"("error in (no error)"=w314, "Data"=w316, "Command"=w315) -> ("error out"=w307:errorcluster, "Data String"=w313:string)  [unwired: 7 in]
        n128 = Unbundle By Name(w312) -> ("Streaming Cfg-Cmds"=w311:T9[], "Streaming Constant Commands"=w310:string[])
        n129 = call "SRV_Sensor PARSE_##R.vi"("Return Data"=w313) -> ("Constant Command"=w309:string, "Value"=w308:dbl)  [unwired: 13 in]
        n130 = call "SRV_Build Sensor-Value Cluster.vi"("Cfg-Cmds"=w311, "Constant Commands"=w310, "Constant Command"=w309, "Value"=w308, "error in (no error)"=w307) -> ("Array of Sensor-Value Cluster"=w301:T11[], "error out"=w304:errorcluster)  [unwired: 9 in]
        n131 = call "SRV_Queue_Enqueue Element at Front.vi"("error in (no error)"=w304, "Data"=w301, "Command"="Update Sensor Value", "Command-Data Queue"=w306) -> ("error out"=w303:errorcluster, "Command-Data Queue out"=w305:refnum<queue>)  [unwired: 5 in, 1 out]
      }
      frame #12 {
        n132 = Variant To Data(error in=w324, Variant=w323, type=T11[] [] ("Array of Sensor-Value Cluster")) -> (error out=w319:errorcluster, data=w320:T11[])
        n133 = Unbundle By Name(w322) -> ("Sensor View refs"=w321:T2)
        n134 = for {
          tunnel: w321 -> [w335]
          tunnel: w320 -> [w334] mode=indexing
          shift-right: [w329] -> w318
          shift-left: w319 -> [w332]
          n135 = Unbundle By Name(w334) -> ("Sensor Name"=w333:T7, "Value"=w327:dbl)
          n136 = call "SRV_Get Sensor View ref From Selection.vi"("Sensor View refs"=w335, "Sensor View"=w333, "error in (no error)"=w332) -> ("Boolean ref?"=w328:bool, "Selected ref"=w331:refnum<vi>, "error out"=w330:errorcluster)  [unwired: 8 in, 2 out]
          n137 = case "Is Boolean ref?" shown="True" w328 {
            tunnel: w327 -> [w337 w340]
            tunnel: [w336 w338] -> w326
            frame #0 {
              n138 = To Variant(anything=w337) -> (Variant=w336:variant)
            }
            frame #1 {
              n139 = call "SRV_Is Not Equal to Zero.vi"("Numeric (DBL)"=w340) -> ("Not Zero"=w339:bool)  [unwired: 14 in]
              n140 = To Variant(anything=w339) -> (Variant=w338:variant)
            }
          }
          n141 = property class="Ctl"(reference=w331, error in=w330, "Value"=w326) -> (error out=w329:errorcluster)  [unwired: 1 out]
        }
      }
      frame #13 {
        # "generates an error with a useful message when an undefined state is requested"
        n142 = Format Into String(format string="Developer Error: the case \"%s\" is undefined.", w345) -> (resulting string=w341:string)  [unwired: 2 in, 1 out]
        n143 = call "SRV_Generate Error.vi"("Message"=w341, "error in (no error)"=w343) -> ("error out"=w342:errorcluster)  [unwired: 13 in]
      }
      frame #14 {
        w348 = T12 1 items=["no dialog", "OK message", "continue or stop message", "OK message + warnings", "continue/stop + warnings"] ("type of dialog (OK msg:1)")
        # "Use Default If Unwired because in the other cases empty string is the same as wiring \"Error\" in the Error-State Controller VI"
        # "append the recent command history to the error souce string"
        n144 = call "SRV_Format Command History String.vi"("Command History"=w355) -> ("Command History String"=w351:string)  [unwired: 14 in]
        n145 = call "SRV_Append to New Error Source String.vi"("Message String to append"=w351, "Error In (no error)"=w352) -> ("error out"=w350:errorcluster)  [unwired: 13 in]
        n146 = call <vilib>:"General Error Handler.vi"("type of dialog (OK msg:1)"=w348, "error in (no error)"=w350) -> ("error out"=w349:errorcluster)  [unwired: 9 in, 4 out]
      }
      frame #15 {
        n147 = call "SRV_VIG_Sensor View Tab Open.vi"("Sensor View Tab Open"=FALSE, "Method (Get)"=enum16{"Get", "Set"}."Set") -> ("error out"=w360:errorcluster)  [unwired: 12 in, 1 out]
        n148 = Unbundle By Name(w365) -> ("SRV ref"=w362:refnum<k5>, "Streaming Cfg-Cmds"=w364:T9[])
        n149 = call "SRV_Sensor Streaming Sensors Off.vi"("Previous Streaming Cfg-Cmds"=w364, "error in (no error)"=w360) -> ("Streaming Cfg-Cmds OFF"=w361:T9[], "error out"=w363:errorcluster)  [unwired: 12 in]
        n150 = call "SRV_Write Sensor Commands.vi"("SRV In"=w362, "Sensor Cfg-Commands"=w361, "error in (no error)"=w363) -> ("error out"=w357:errorcluster)  [unwired: 11 in, 1 out]
        n151 = Select(t=w359, s=w359, f=w357) -> (s? t:f=w358:errorcluster)
      }
    }
    n152 = call "SRV_Command Queue Error-State Controller.vi"("error in (no error)"=w104, "Error Command"=w98, "Command-Data Queue"=w102) -> ("error out"=w103:errorcluster, "Command-Data Queue out"=w101:refnum<queue>)  [unwired: 7 in]
  }
  n153 = while {
    shift-right: [w374] -> w85
    shift-left: w87 -> [w375]
    tunnel: w4 -> [w373]
    tunnel: w88 -> [w372]
    tunnel: [w371] -> w86
    stop <- w370 stop-if-true
    n154 = event shown="[0] \"Poll\": Value Change" {
      selector: w372 -> [_ _]
      dyn-events: [_ _] -> w371
      timeout: _ -> [_ _]
      tunnel: w375 -> [w377 w381]
      tunnel: [w378 w381] -> w374
      tunnel: w373 -> [w376 _]
      tunnel: [_ TRUE] -> w370
      event #0 {
        n155 = event-data() -> ()  [unwired: 1 in, 5 out]
        n156 = call "SRV_Queue_Enqueue Element.vi"("error in (no error)"=w377, "Command"="Poll", "Command-Data Queue"=w376) -> ("error out"=w378:errorcluster)  [unwired: 6 in, 2 out]
      }
      event #1 {
        n157 = event-data() -> ()  [unwired: 1 in, 1 out]
      }
    }
  }
  n158 = Unregister For Events(event registration refnum=w86, error in=w85) -> (error out=w75:errorcluster)
  n159 = Unbundle By Name(w80) -> ("Make All Visible"=w1:bool, "This VI ref"=w15:refnum<vi>, "user event"=w79:refnum<user-event>)
  n160 = Release Queue(queue=w83, force destroy? (F)=TRUE, error in (no error)=w84) -> (error out=w78:errorcluster)  [unwired: 2 out]
  n161 = call "SRV_Generate User Exit Event.vi"("error in (no error)"=w78, "User Exit Event"=w79) -> ("error out"=w76:errorcluster, "User Exit Event out"=w77:refnum<user-event>)  [unwired: 8 in]
  n162 = Build Array(w76, w75) -> (w71:errorcluster[])
  n163 = call <vilib>:"Merge Errors.vi"("error array in"=w71) -> ("error out"=w74:errorcluster)  [unwired: 6 in]
  n164 = Destroy User Event(user event=w77, error in=w74) -> (error out=w17:errorcluster)
  n165 = flat-sequence {
    tunnel: w17 -> [w386]
    tunnel: [w386] -> w16
    tunnel: w15 -> [w385]
    tunnel: w1 -> [w382]
    frame #0 {
      n166 = Compound Arithmetic op=AND(TRUE, invert w382) -> (w384:bool)
      n167 = case shown="True" w384 {
        tunnel: w385 -> [_ w388]
        frame #0 {
        }
        frame #1 {
          n168 = invoke class="VI" method="FP.Close"(reference=w388) -> (error out=w387:errorcluster)  [unwired: 2 in, 2 out]
          n169 = call <vilib>:"Clear Errors.vi"("error in (no error)"=w387) -> ()  [unwired: 6 in, 1 out]
        }
      }
    }
  }
  "error out" <- w16
